vi "Data Files Setup.vi"(8 "error in (no error)":errorcluster, 11 "Data Directory":path=path "C:/Users/plane/Desktop/LabVIEW/Data") -> (0 "error out":errorcluster, 1 "Log File Ref":refnum<file>, 2 "Reduced Data File Ref":refnum<file>, 3 "Raw Data File Ref":refnum<file>)   [LabVIEW 2013]
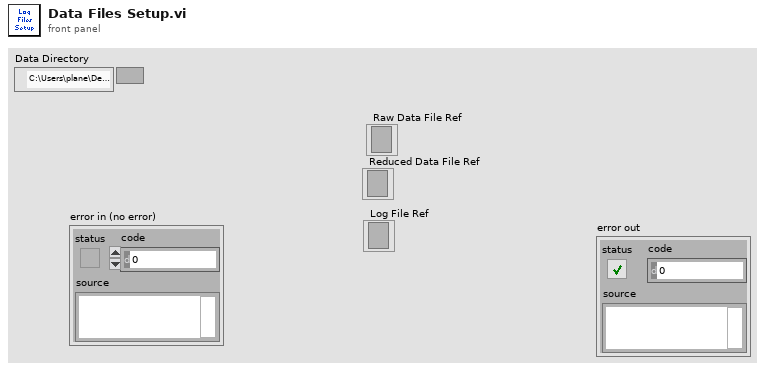
[diagram p1: front panel]
types:
  T1 = enum16{"open", "replace", "create", "open or create", "replace or create", "replace or create with confirmation"}
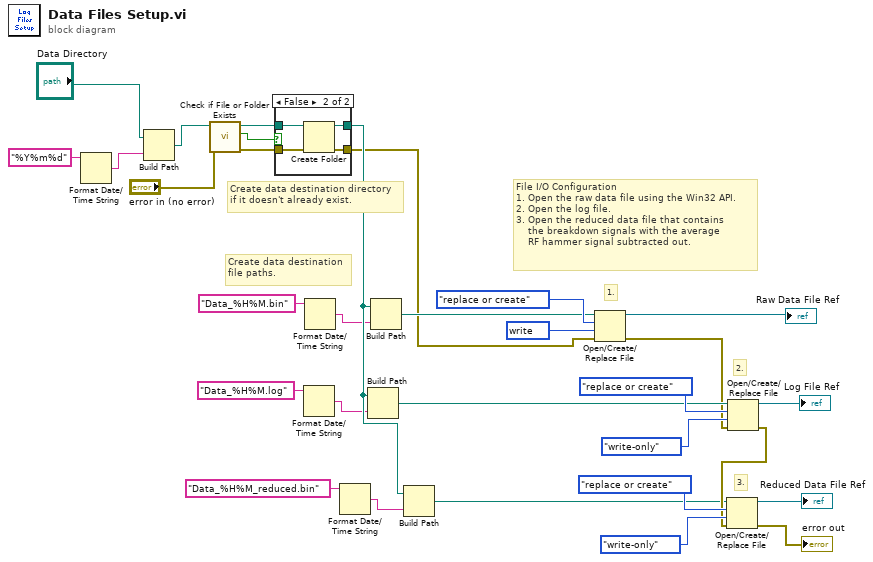
[diagram p0: block diagram]
diagram:
  w21 = u32 1073741824 items=["read"=2147483648, "write"=1073741824, "read & write"=3221225472, "execute"=536870912, "all"=268435456] ("desired access (read & write)")
  # "Create data destination\nfile paths."
  # "Create data destination directory\nif it doesn't already exist."
  # "1."
  # "File I/O Configuration\n1. Open the raw data file using the Win32 API.\n2. Open the log file.\n3. Open the reduced data file that contains\n    the breakdown signals with the average\n    RF hammer signal subtracted out."
  # "3."
  # "2."
  n1 = Format Date/Time String(time format string (%c)="%Y%m%d") -> (date/time string=w16:string)  [unwired: 2 in]
  n2 = Build Path(base path="Data Directory", name or relative path=w16) -> (appended path=w14:path)
  n3 = call <vilib>:"Check if File or Folder Exists.vi"("error in (no error)"="error in (no error)", "path"=w14) -> ("error out"=w11:errorcluster, "file or folder exists?"=w12:bool, "dup path"=w13:path)  [unwired: 7 in]
  n4 = case shown="False" w12 {
    tunnel: w13 -> [w33 w37]
    tunnel: [w33 w36] -> w8
    tunnel: w11 -> [w32 w35]
    tunnel: [w32 w34] -> w1
    frame True {
    }
    frame False {
      n5 = Create Folder(path (use dialog)=w37, error in=w35) -> (created path=w36:path, error out=w34:errorcluster)  [unwired: 1 in, 1 out]
    }
  }
  n6 = Format Date/Time String(time format string (%c)="Data_%H%M.log") -> (date/time string=w5:string)  [unwired: 2 in]
  n7 = Format Date/Time String(time format string (%c)="Data_%H%M.bin") -> (date/time string=w7:string)  [unwired: 2 in]
  n8 = Format Date/Time String(time format string (%c)="Data_%H%M_reduced.bin") -> (date/time string=w3:string)  [unwired: 2 in]
  n9 = Build Path(base path=w8, name or relative path=w5) -> (appended path=w24:path)
  n10 = Build Path(base path=w8, name or relative path=w7) -> (appended path=w18:path)
  n11 = Build Path(base path=w8, name or relative path=w3) -> (appended path=w23:path)
  n12 = Open/Create/Replace File(file path (use dialog)=w18, error in=w1, operation (0:open)=T1."replace or create", access (0:read/write)=w21) -> (refnum out=→"Raw Data File Ref":refnum<file>, error out=w19:errorcluster)  [unwired: 2 in, 1 out]
  n13 = Open/Create/Replace File(file path (use dialog)=w24, error in=w19, operation (0:open)=T1."replace or create", access (0:read/write)=enum16{"read/write", "read-only", "write-only"}."write-only") -> (refnum out=→"Log File Ref":refnum<file>, error out=w25:errorcluster)  [unwired: 2 in, 1 out]
  n14 = Open/Create/Replace File(file path (use dialog)=w23, error in=w25, operation (0:open)=T1."replace or create", access (0:read/write)=enum16{"read/write", "read-only", "write-only"}."write-only") -> (refnum out=→"Reduced Data File Ref":refnum<file>, error out=→"error out":errorcluster)  [unwired: 2 in, 1 out]
